vi "updateWaypoints.vi"(8 "error in (no error)":errorcluster, 11 "StationKeeping in":refnum<class "StationKeeping.lvclass">) -> (0 "error out":errorcluster, 3 "StationKeeping out":refnum<class "StationKeeping.lvclass">)   [LabVIEW 2011, in "StationKeeping.lvclass"]
doc: "Handles the 3 phases of the station keeping mission, while it is in progress. First, it checks if the mission should be started, by checking if the robot is in the station or not. If not, the start time is reset for the mission.\nIf so, using a timer, it checks which phase of the mission it is in. In the first phase, it calls \"station_keeping_waypoints.vi\" and adds waypoints to the waypoints array from a pattern in that VI. In the second phase, it adds waypoints along the edge of the boundary. These are 7 meters from the corners regardless of station size. In the third phase, it adds a waypoint outside the boundary (w/out a No-Sail Zone)\n\nThe purpose of the Local Variable \"Phase\" is to check when the phase is changing. The first time a phase changes, the \"current waypoint\" global is updated, in order to check off unecessary waypoints."
uses:
  StationKeeping.lvclass
  StationKeeping.lvclass/StationKeeping.ctl
  2 Globals/2 Global.vi
  Waypoint/Waypoint.lvclass
panel:
  out "Phase":dbl
  out "Time Elapsed":dbl
  out "Time Remaining":dbl
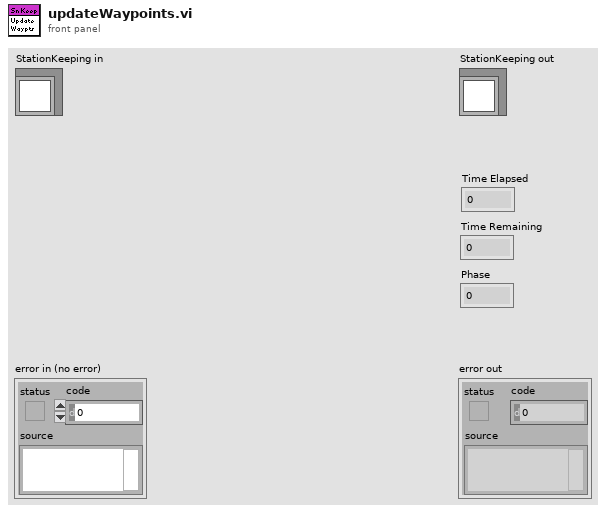
[diagram p1: front panel]
types:
  T1 = typedef "UTM Location.ctl" = cluster{"UTM Zone":dbl, "Hemisphere":enum16{"North", "South"}, "East":dbl, "North":dbl}
  T2 = typedef "Waypoints List.ctl" = refnum<class "Waypoint.lvclass">[]
  T3 = typedef "UTM Circle.ctl" = cluster{"UTM Zone":dbl, "Hemisphere":enum16{"North", "South"}, "East":dbl, "North":dbl, "Radius":dbl}
  T4 = typedef "Current Waypoint.ctl" = i32
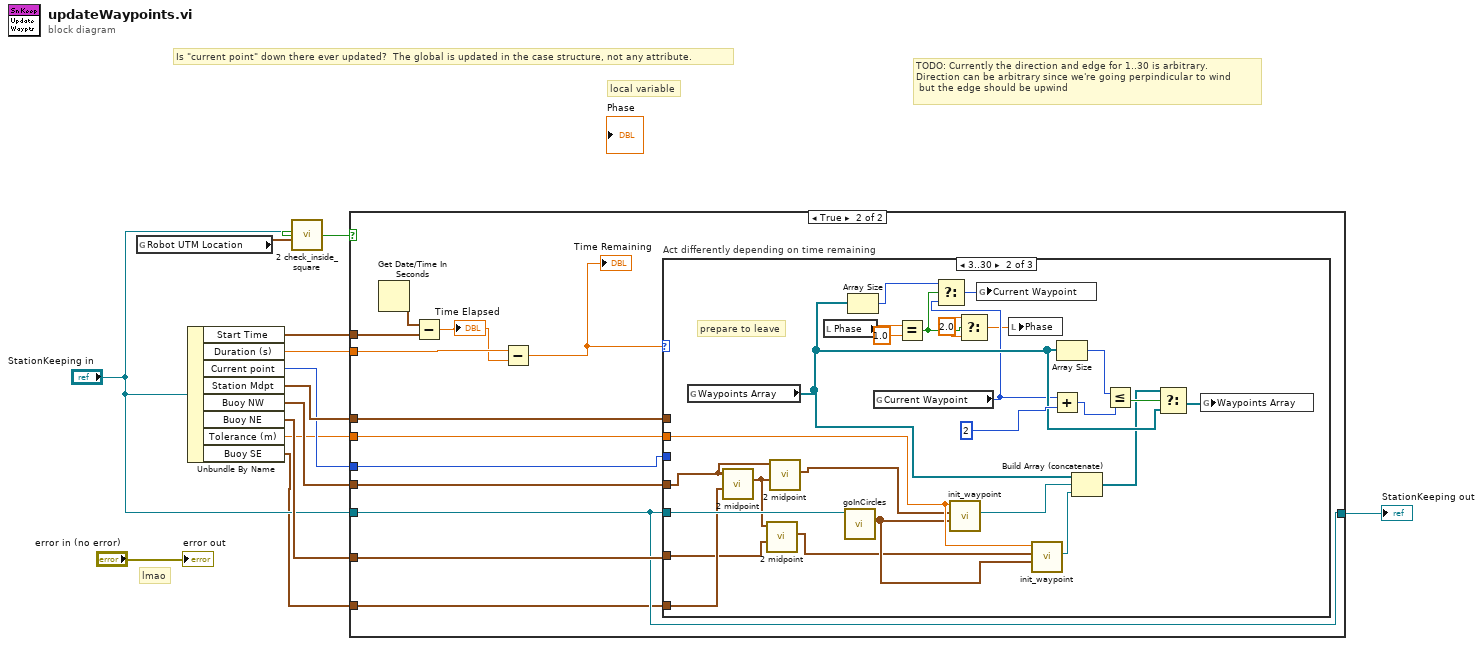
[diagram p0: block diagram]
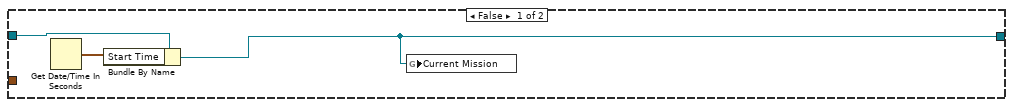
[diagram p2: hidden frame]
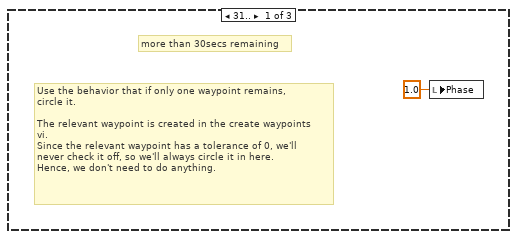
[diagram p3: hidden frame]
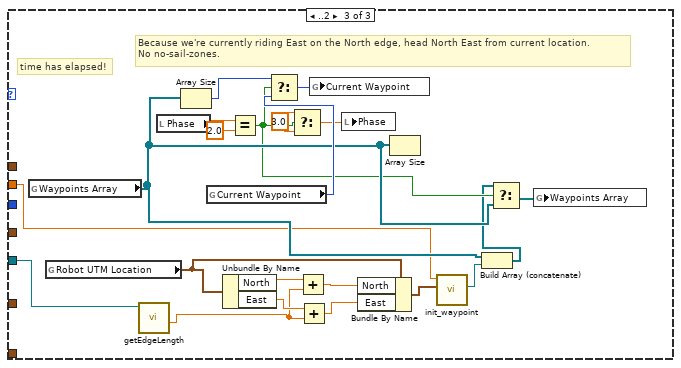
[diagram p4: hidden frame]
diagram:
  # "local variable"
  # "TODO: Currently the direction and edge for 1..30 is arbitrary.  \nDirection can be arbitrary since we're going perpindicular to wind\n but the edge should be upwind"
  # "Is \"current point\" down there ever updated?  The global is updated in the case structure, not any attribute."
  # "lmao"
  n1 = global read "2 Global.vi" "Robot UTM Location"() -> (w2:T1)
  n2 = Unbundle By Name("StationKeeping in") -> ("Start Time"=w13:timestamp, "Duration (s)"=w12:dbl, "Current point"=w7:i32, "Station Mdpt"=w11:T1, "Buoy NW"=w9:T1, "Buoy NE"=w8:T1, "Tolerance (m)"=w6:dbl, "Buoy SE"=w1:T1)
  n3 = call "2 check_inside_square.vi"("UTM Location"=w2, "StationKeeping.lvclass"="StationKeeping in") -> ("In Square?"=w4:bool)  [unwired: 9 in]
  n4 = case shown="True" w4 {
    tunnel: w13 -> [_ w27]
    tunnel: w12 -> [_ w26]
    tunnel: w11 -> [_ w24]
    tunnel: w9 -> [_ w22]
    tunnel: w8 -> [_ w21]
    tunnel: w7 -> [_ w20]
    tunnel: w6 -> [_ w19]
    tunnel: "StationKeeping in" -> [w15 w18]
    tunnel: [w14 w18] -> w5
    tunnel: w1 -> [_ w17]
    frame False {
      n5 = Get Date/Time In Seconds() -> (seconds since 1Jan1904=w16:timestamp)
      n6 = Bundle By Name(cluster=w15, "Start Time"=w16) -> (w14:refnum<class "StationKeeping.lvclass">)
      n7 = global write "2 Global.vi" "Current Mission"(w14) -> ()
    }
    frame True {
      n8 = Get Date/Time In Seconds() -> (seconds since 1Jan1904=w28:timestamp)
      n9 = Subtract(x=w28, y=w27) -> (x-y=w25:dbl)
      "Time Elapsed" <- w25
      n10 = Subtract(x=w26, y=w25) -> (x-y=w23:dbl)
      "Time Remaining" <- w23
      n11 = case "Act differently depending on time remaining" shown="3..30" w23 {
        tunnel: w20 -> [_ _ _]
        tunnel: w24 -> [_ _ _]
        tunnel: w18 -> [_ w36 w58]
        tunnel: w22 -> [_ w35 _]
        tunnel: w21 -> [_ w30 _]
        tunnel: w19 -> [_ w40 w56]
        tunnel: w17 -> [_ w32 _]
        frame 31.. {
          # "Use the behavior that if only one waypoint remains,\ncircle it.\n\nThe relevant waypoint is created in the create waypoints\nvi.\nSince the relevant waypoint has a tolerance of 0, we'll\nnever check it off, so we'll always circle it in here.\nHence, we don't need to do anything."
          # "more than 30secs remaining"
          n12 = local write "Phase"(1.0 ("Phase")) -> ()
        }
        frame 3..30 {
          w41 = 2.0 ("y")
          # "prepare to leave"
          n13 = global read "2 Global.vi" "Waypoints Array"() -> (w50:T2)
          n14 = call "2 midpoint.vi"("UTM 2"=w32, "UTM 1"=w35) -> ("Midpoint"=w33:T1)  [unwired: 8 in, 1 out]
          n15 = call "2 midpoint.vi"("UTM 2"=w30, "UTM 1"=w33) -> ("Midpoint"=w31:T1)  [unwired: 8 in, 1 out]
          n16 = call "2 midpoint.vi"("UTM 2"=w33, "UTM 1"=w35) -> ("Midpoint"=w34:T1)  [unwired: 8 in, 1 out]
          n17 = local read "Phase"() -> (w47:dbl)
          n18 = call "goInCircles.vi"("StationKeeping in"=w36) -> ("No Sail Circles"=w39:T3[])  [unwired: 8 in, 2 out]
          n19 = Array Size(array=w50) -> (size(s)=w45:i32)
          n20 = global read "2 Global.vi" "Current Waypoint"() -> (w44:T4)
          n21 = Equal?(x=w47, y=1.0) -> (x = y?=w42:bool)
          n22 = Select(t=w45, s=w42, f=w44) -> (s? t:f=w48:T4)
          n23 = call "init_waypoint.vi"("No Sail Circles"=w39, "Coords"=w34, "Tolerance (m)"=w40) -> ("Waypoint Out"=w55:refnum<class "Waypoint.lvclass">)  [unwired: 8 in]
          n24 = Select(t=w41, s=w42, f=w41) -> (s? t:f=w43:dbl)
          n25 = global write "2 Global.vi" "Current Waypoint"(w48) -> ()
          n26 = local write "Phase"(w43) -> ()
          n27 = call "init_waypoint.vi"("No Sail Circles"=w39, "Coords"=w31, "Tolerance (m)"=w40) -> ("Waypoint Out"=w54:refnum<class "Waypoint.lvclass">)  [unwired: 8 in]
          n28 = Add(x=w44, y=2) -> (x+y=w38:T4)
          n29 = Array Size(array=w50) -> (size(s)=w37:i32)
          n30 = Build Array (concatenate)(w50, w55, w54) -> (w49:T2)
          n31 = Less Or Equal?(x=w37, y=w38) -> (x <= y?=w53:bool)
          n32 = Select(t=w49, s=w53, f=w50) -> (s? t:f=w52:T2)
          n33 = global write "2 Global.vi" "Waypoints Array"(w52) -> ()
        }
        frame ..2 {
          w63 = 3.0 ("y")
          # "time has elapsed!"
          # "Because we're currently riding East on the North edge, head North East from current location.\nNo no-sail-zones."
          n34 = global read "2 Global.vi" "Waypoints Array"() -> (w62:T2)
          n35 = global read "2 Global.vi" "Robot UTM Location"() -> (w73:T1)
          n36 = call "getEdgeLength.vi"("StationKeeping in"=w58) -> ("Edge Length"=w57:dbl)  [unwired: 9 in, 1 out]
          n37 = local read "Phase"() -> (w67:dbl)
          n38 = Array Size(array=w62) -> (size(s)=w59:i32)
          n39 = global read "2 Global.vi" "Current Waypoint"() -> (w65:T4)
          n40 = Unbundle By Name(w73) -> ("North"=w75:dbl, "East"=w76:dbl)
          n41 = Equal?(x=w67, y=2.0) -> (x = y?=w61:bool)
          n42 = Select(t=w59, s=w61, f=w65) -> (s? t:f=w68:T4)
          n43 = Select(t=w63, s=w61, f=w63) -> (s? t:f=w64:dbl)
          n44 = Add(x=w75, y=w57) -> (x+y=w74:dbl)
          n45 = Add(x=w76, y=w57) -> (x+y=w72:dbl)
          n46 = global write "2 Global.vi" "Current Waypoint"(w68) -> ()
          n47 = local write "Phase"(w64) -> ()
          n48 = Bundle By Name(cluster=w73, "North"=w74, "East"=w72) -> (w70:T1)
          n49 = Array Size(array=w62) -> ()  [unwired: 1 out]
          n50 = call "init_waypoint.vi"("Coords"=w70, "Tolerance (m)"=w56) -> ("Waypoint Out"=w71:refnum<class "Waypoint.lvclass">)  [unwired: 9 in]
          n51 = Build Array (concatenate)(w62, w71) -> (w60:T2)
          n52 = Select(t=w60, s=w61, f=w62) -> (s? t:f=w69:T2)
          n53 = global write "2 Global.vi" "Waypoints Array"(w69) -> ()
        }
      }
    }
  }
  "StationKeeping out" <- w5
  "error out" <- "error in (no error)"
